vi "Main.vi"() -> ()   [LabVIEW 2022 SP3]
uses:
  <vilib>/OPCUA/client/Multiple Read Double.vi
  <vilib>/OPCUA/NI OPC UA Client.lvlib
panel:
  out "Name":string
  out "Temperature vs Time":cluster{"Temp":dbl, "Setpoint":dbl}(graph)
  in  "Tab Control":enum32{"OPC", "Readings", "Database"}(tab)=enum."Database"
  in  "OPC URL":string="opc.tcp://DESKTOP-D4R0VU6:49580"
  in  "Temp Node ID":string="ProcessData.Temperature" caption="Process Tempertature Node ID"
  in  "V Node ID":string="ProcessData.ControlVoltage" caption="Control Voltage Node ID"
  in  "Setpoint Node ID":string="ProcessData.Setpoint"
  in  "E_Temp Node ID":string="ProcessData.Environment" caption="Environment Temperature Node ID"
  out "Temp":dbl=29.999979335255162 caption="Process Temperature [Deg C]" format="%.1g"
  out "Setpoint":dbl=30.0 caption="Setpoint Temperature [Deg C]" format="%.1g"
  out "E_Temp":dbl=21.5 caption="Envvironment Temperature [Deg C]"
  out "V":dbl=2.428572184284423 caption="Control Voltage [V]" format="%.2g"
  out "Time Stamp":timestamp=timestamp(3766513438.495935 s since 1904-01-01) format="%<%X\n%x>T"
  in  "ODBC Connection":string="SCADA"
  in  "Ts [s]":dbl=2.0 caption="Data logging interval [s]"
  out "error out":errorcluster
  in  "error in":errorcluster
  in  "Stop Button":bool
  # "Datalogging Module"
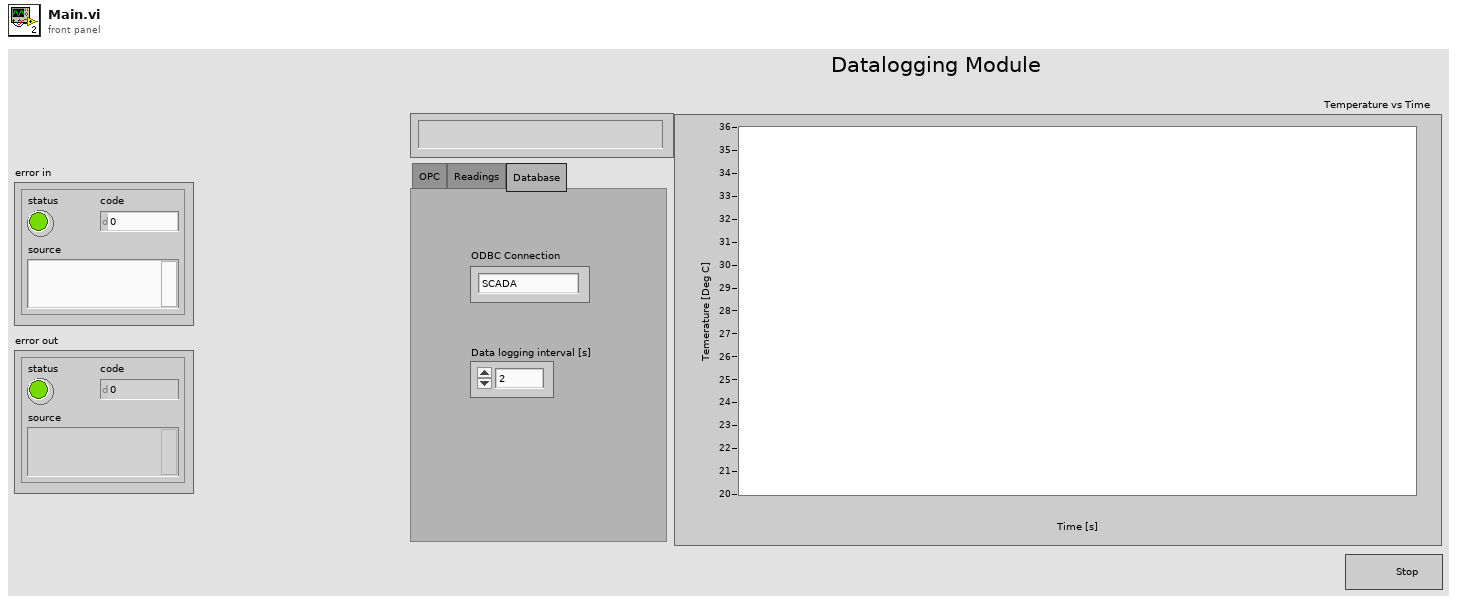
[diagram p1: front panel]
types:
  T1 = cluster{"message mode":enum16{"None", "Sign", "Sign and Encrypt"}, "security":enum16{"Basic256", "Basic128Rsa15"}}
  T2 = typedef "OPC UA Client Refnum.ctl" = refnum<k21>
  T3 = typedef "NodeId.ctl" = string
  T4 = typedef "OPC UA StatusCode.ctl" = u32
  T5 = cluster{"node ID":T3, "value ":dbl, "timestamp":timestamp, "status":T4}[]
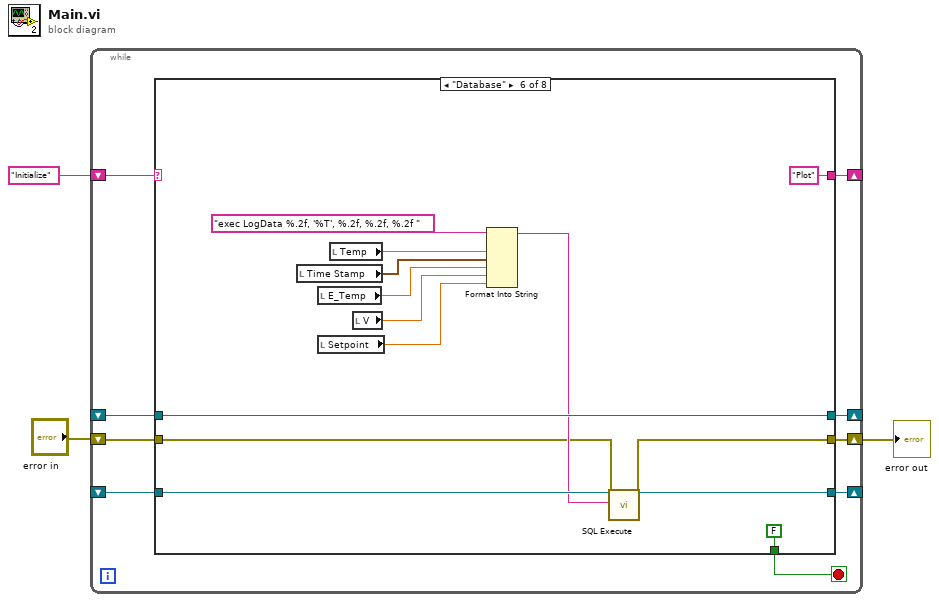
[diagram p0: block diagram]
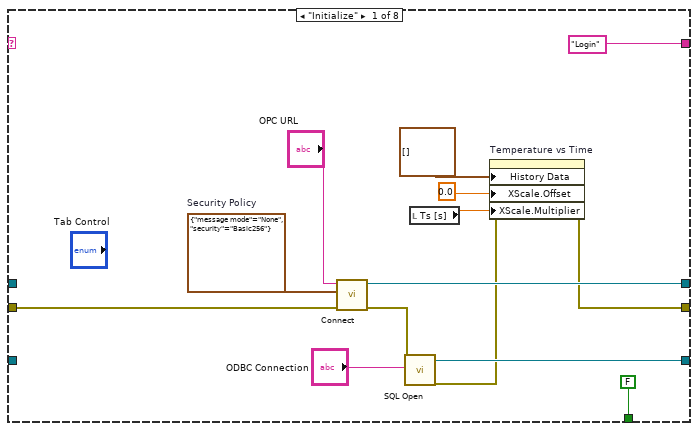
[diagram p2: hidden frame]
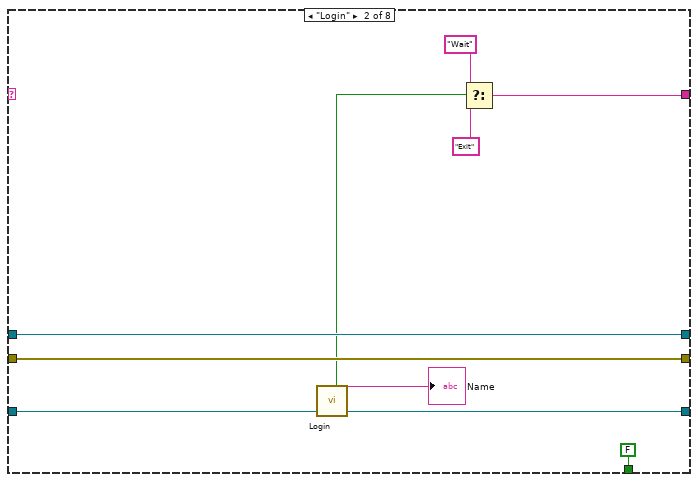
[diagram p3: hidden frame]
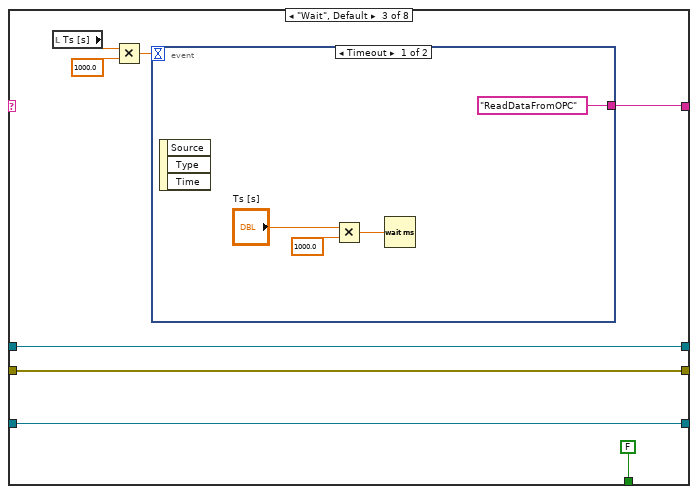
[diagram p4: hidden frame]
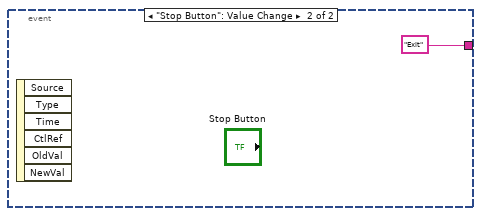
[diagram p5: hidden frame]
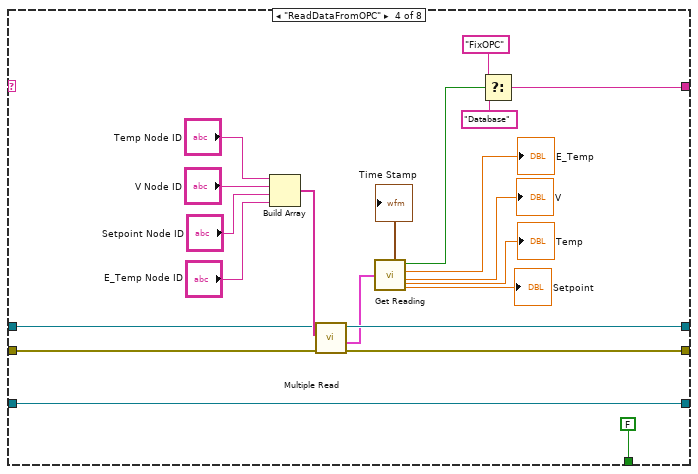
[diagram p6: hidden frame]
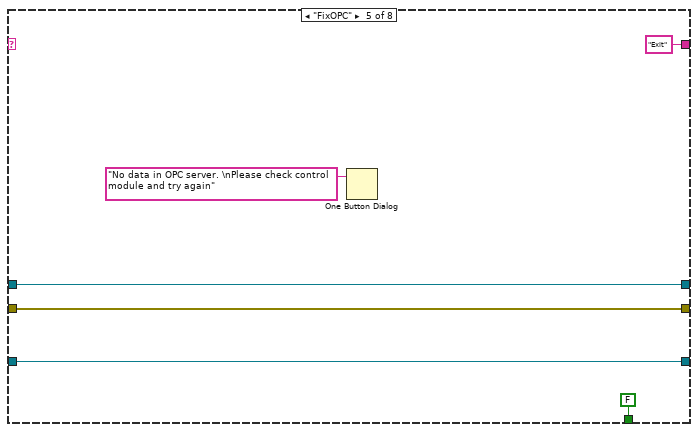
[diagram p7: hidden frame]
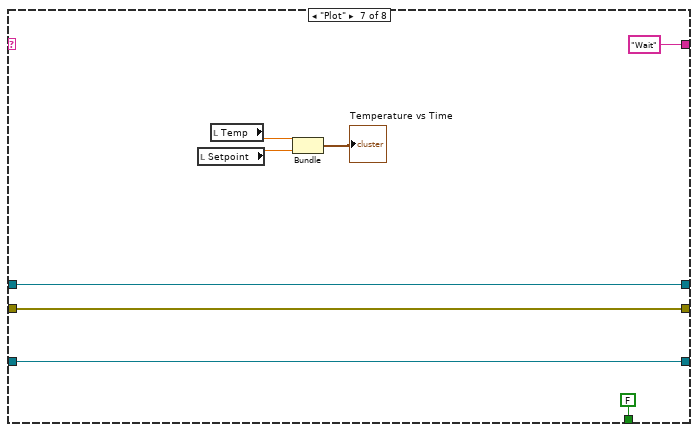
[diagram p8: hidden frame]
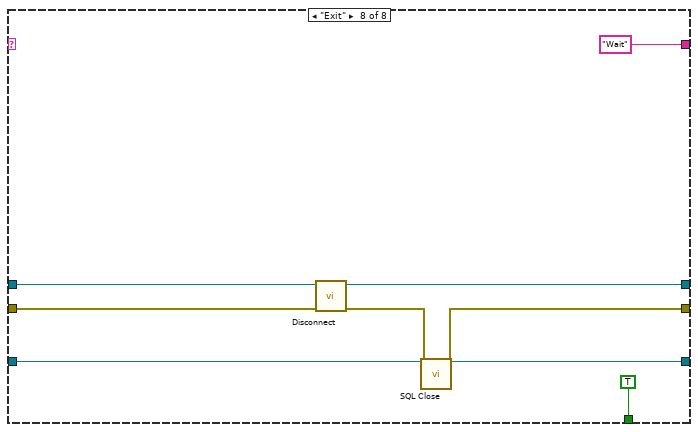
[diagram p9: hidden frame]
diagram:
  n1 = while {
    shift-right: [w11] -> _
    shift-left: "Initialize" -> [w12]
    shift-right: [w8] -> w1
    shift-left: "error in" -> [w9]
    shift-right: [w7] -> _
    shift-left: _ -> [w6]
    shift-right: [w5] -> _
    shift-left: _ -> [w4]
    stop <- w10 stop-if-true
    n2 = case shown="\"Database\"" w12 {
      tunnel: ["Login" w28 w44 w50 "Exit" ("t") "Plot" "Wait" "Wait"] -> w11
      tunnel: [FALSE FALSE FALSE FALSE FALSE FALSE FALSE TRUE] -> w10
      tunnel: w9 -> [w23 w35 w40 w69 w73 w78 w96 w105]
      tunnel: [w17 w35 w40 w68 w73 w77 w96 w101] -> w8
      tunnel: [w21 w34 w38 w63 w74 w89 w97 w102] -> w7
      tunnel: w6 -> [_ w34 w38 w62 w74 w89 w97 w102]
      tunnel: [w20 w32 w37 w54 w72 w87 w95 w99] -> w5
      tunnel: w4 -> [_ w33 w37 w54 w72 w86 w95 w99]
      frame "Initialize" {
        w25 = T1 {"message mode"=enum."None", "security"=enum."Basic256"}  # Security Policy
        n3 = call <vilib>:"Connect.vi"("error in (no error)"=w23, "security policy"=w25, "server endpoint URL"="OPC URL") -> ("error out"=w19:errorcluster, "OPC UA client refnum out"=w21:T2)  [unwired: 6 in, 1 out]
        n4 = call <vilib>:"SQL Open.vi"("ConnectionString In"="ODBC Connection", "Error in (no error)"=w19) -> ("Connection Out"=w20:refnum<k7>, "Error out"=w16:errorcluster)  [unwired: 16 in]
        n5 = local read "Ts [s]"() -> (w13:dbl)
        n6 = property on="Temperature vs Time" class="WFChart (strict)"(error in=w16, "History Data"=cluster{"Temp":dbl, "Setpoint":dbl}[] [], "XScale.Offset"=0.0 ("X Scale.Offset and Multiplier:Offset"), "XScale.Multiplier"=w13) -> (error out=w17:errorcluster)  [unwired: 1 in, 1 out]
      }
      frame "Login" {
        n7 = call "Login.vi"("Connection In"=w33) -> ("Not empty?"=w30:bool, "Connection Out"=w32:refnum<k7>, "Name"=→"Name":string)  [unwired: 1 in, 3 out]
        n8 = Select(t="Wait", s=w30, f="Exit") -> (s? t:f=w28:string)
      }
      frame "Wait", Default {
        n9 = local read "Ts [s]"() -> (w41:dbl)
        n10 = Multiply(x=w41, y=1000.0) -> (x*y=w43:dbl)
        n11 = event shown="[0] Timeout" {
          selector: _ -> [_ _]
          dyn-events: _ -> [_ _]
          timeout: w43 -> [_ _]
          tunnel: ["ReadDataFromOPC" "Exit"] -> w44
          event Timeout {
            n12 = event-data() -> ()  [unwired: 1 in, 3 out]
            n13 = Multiply(x="Ts [s]", y=1000.0) -> (x*y=w47:dbl)
            n14 = Wait (ms)(milliseconds to wait=w47) -> ()  [unwired: 1 out]
          }
          event "Stop Button": Value Change {
            n15 = event-data() -> ()  [unwired: 1 in, 6 out]
          }
        }
      }
      frame "ReadDataFromOPC" {
        n16 = Build Array "Build Array"("Temp Node ID", "V Node ID", "Setpoint Node ID", "E_Temp Node ID") -> (w64:string[])
        n17 = call-poly <vilib>:"Multiple Read.vi"("error in (no error)"=w69, "node IDs"=w64, "OPC UA client refnum in"=w62) -> ("error out"=w68:errorcluster, "results"=w60:T5, "OPC UA client refnum out"=w63:T2)  [unwired: 5 in, 1 out]
        n18 = call "Get Reading.vi"("results"=w60) -> ("Time Stamp"=→"Time Stamp":timestamp, "Process Temperature [Deg C]"=→"Temp":dbl, "empty?"=w53:bool, "Environment Temperature [Deg C]"=→"E_Temp":dbl, "Control Voltage [V]"=→"V":dbl, "Setpoint [Deg C]"=→"Setpoint":dbl)
        n19 = Select(t="FixOPC", s=w53, f="Database") -> (s? t:f=w50:string)
      }
      frame "FixOPC" {
        n20 = One Button Dialog(message="No data in OPC server. \nPlease check control module and try again") -> ()  [unwired: 1 in, 1 out]
      }
      frame "Database" {
        n21 = local read "Time Stamp"() -> (w83:timestamp)
        n22 = local read "E_Temp"() -> (w82:dbl)
        n23 = local read "Setpoint"() -> (w80:dbl)
        n24 = local read "Temp"() -> (w85:dbl)
        n25 = local read "V"() -> (w81:dbl)
        n26 = Format Into String "Format Into String"(format string="exec LogData %.2f, '%T', %.2f, %.2f, %.2f ", w85, w83, w82, w81, w80) -> (resulting string=w79:string)  [unwired: 2 in, 1 out]
        n27 = call <vilib>:"SQL Execute.vi"("Connection In"=w86, "SQL Query"=w79, "Error in (no error)"=w78) -> ("Connection Out"=w87:refnum<k7>, "Error out"=w77:errorcluster)  [unwired: 15 in]
      }
      frame "Plot" {
        n28 = local read "Setpoint"() -> (w91:dbl)
        n29 = local read "Temp"() -> (w93:dbl)
        n30 = Bundle("Temp"=w93, "Setpoint"=w91) -> (→"Temperature vs Time":cluster{"Temp":dbl, "Setpoint":dbl})  [unwired: 1 in]
      }
      frame "Exit" {
        n31 = call <vilib>:"Disconnect.vi"("error in (no error)"=w105, "OPC UA client refnum in"=w102) -> ("error out"=w100:errorcluster)  [unwired: 9 in]
        n32 = call <vilib>:"SQL Close.vi"("Connection In"=w99, "Error in (no error)"=w100) -> ("Error out"=w101:errorcluster)  [unwired: 17 in]
      }
    }
  }
  "error out" <- w1
